vi "Update Cycles.vi"(8 "error in (no error)":errorcluster, 11 "Tamagotchi Full Actor in":refnum<class "Tamagotchi Full Actor.lvclass">) -> (0 "error out":errorcluster, 3 "Tamagotchi Full Actor out":refnum<class "Tamagotchi Full Actor.lvclass">)   [LabVIEW 2026, in "Tamagotchi Full Actor.lvclass"]
uses:
  Tamagotchi Full Actor.lvclass
  Tamagotchi Full Actor.lvclass/Tamagotchi Full Actor.ctl
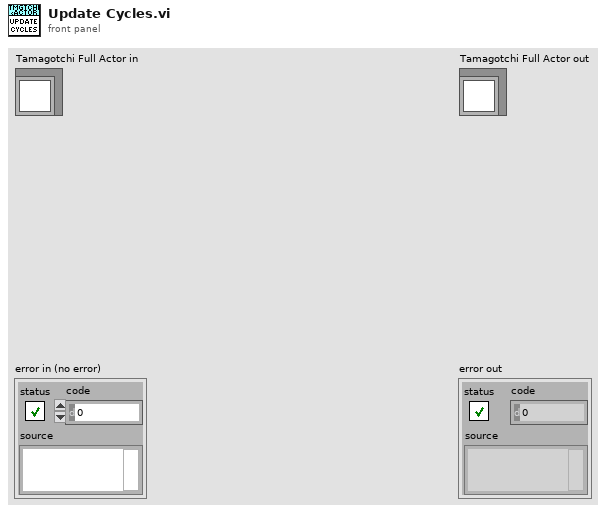
[diagram p1: front panel]
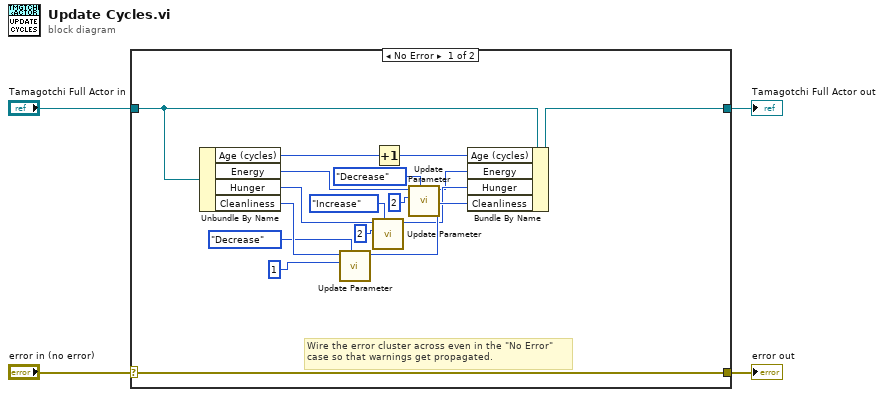
[diagram p0: block diagram]
diagram:
  n1 = case shown="No Error" "error in (no error)" {
    selector: "error in (no error)" -> [w21 w23]
    tunnel: [w21 w23] -> w3
    tunnel: [w5 w22] -> w1
    tunnel: "Tamagotchi Full Actor in" -> [w6 w22]
    frame No Error {
      # "Wire the error cluster across even in the \"No Error\"\ncase so that warnings get propagated."
      n2 = Unbundle By Name(w6) -> ("Age (cycles)"=w13:u32, "Energy"=w15:i16, "Hunger"=w17:i16, "Cleanliness"=w19:i16)
      n3 = call "Update Parameter.vi"("Action"=enum16{"Increase", "Decrease"}."Decrease", "Modifier"=i16 1, "Parameter"=w19) -> ("New Value"=w20:i16)  [unwired: 8 in]
      n4 = call "Update Parameter.vi"("Action"=enum16{"Increase", "Decrease"}."Increase", "Modifier"=i16 2, "Parameter"=w17) -> ("New Value"=w18:i16)  [unwired: 8 in]
      n5 = Increment(x=w13) -> (x+1=w14:u32)
      n6 = call "Update Parameter.vi"("Action"=enum16{"Increase", "Decrease"}."Decrease", "Modifier"=i16 2, "Parameter"=w15) -> ("New Value"=w16:i16)  [unwired: 8 in]
      n7 = Bundle By Name(cluster=w6, "Age (cycles)"=w14, "Energy"=w16, "Hunger"=w18, "Cleanliness"=w20) -> (w5:refnum<class "Tamagotchi Full Actor.lvclass">)
    }
    frame Error {
    }
  }
  "error out" <- w3
  "Tamagotchi Full Actor out" <- w1
